vi "Read Target ESI Files.vi"(8 "error in":errorcluster) -> (0 "error out":errorcluster)   [LabVIEW 2019, in "SEECD System Explorer.lvlib"]
uses:
  SEECD System Explorer.lvlib
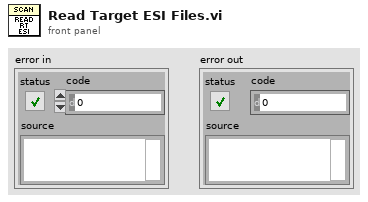
[diagram p1: front panel]
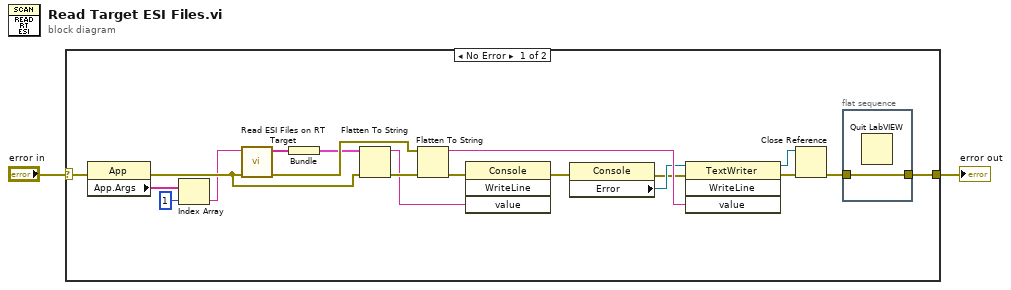
[diagram p0: block diagram]
diagram:
  n1 = case shown="No Error" "error in" {
    selector: "error in" -> [w20 w23]
    tunnel: [w18 w23] -> w2
    frame No Error {
      n2 = property class="App"(error in=w20) -> (error out=w4:errorcluster, "App.Args"=w21:string[])  [unwired: 1 in, 1 out]
      n3 = Index Array(array=w21, index=1) -> (element=w3:string)
      n4 = call "Read ESI Files on RT Target.vi"("error in"=w4, "Target IP"=w3) -> ("error out"=w8:errorcluster, "Existing Target Profiles"=w6:string[])  [unwired: 8 in]
      n5 = Bundle("Existing Target Profiles"=w6) -> (w5:cluster{"Existing Target Profiles":string[]})  [unwired: 1 in]
      n6 = Flatten To String(anything=w5, error in (no error)=w4) -> (data string=w15:string, error out=w17:errorcluster)  [unwired: 2 in, 1 out]
      n7 = Flatten To String(anything=w8, error in (no error)=w17) -> (data string=w14:string, error out=w16:errorcluster)  [unwired: 2 in, 1 out]
      n8 = invoke class="Console" method="WriteLine"(error in=w16, "value"=w15) -> (error out=w7:errorcluster)  [unwired: 2 in, 3 out]
      n9 = property class="Console"(error in=w7) -> (error out=w9:errorcluster, "Error"=w13:refnum<k24>)  [unwired: 1 in, 1 out]
      n10 = invoke class="TextWriter" method="WriteLine"(reference=w13, error in=w9, "value"=w14) -> (reference out=w11:refnum<k24>, error out=w12:errorcluster)  [unwired: 1 in, 2 out]
      n11 = Close Reference(reference=w11, error in (no error)=w12) -> (error out=w10:errorcluster)
      n12 = flat-sequence {
        tunnel: w10 -> [w22]
        tunnel: [w22] -> w18
        frame #0 {
          n13 = Quit LabVIEW() -> ()  [unwired: 1 in]
        }
      }
    }
    frame Error {
    }
  }
  "error out" <- w2
